vi "zad1.vi"() -> ()   [LabVIEW 2017]
panel:
  out "result string":string[](array[string])
  in  "tekst":string
  in  "litera":string
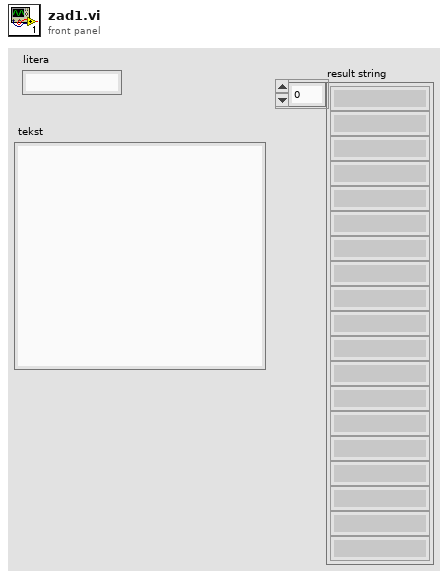
[diagram p1: front panel]
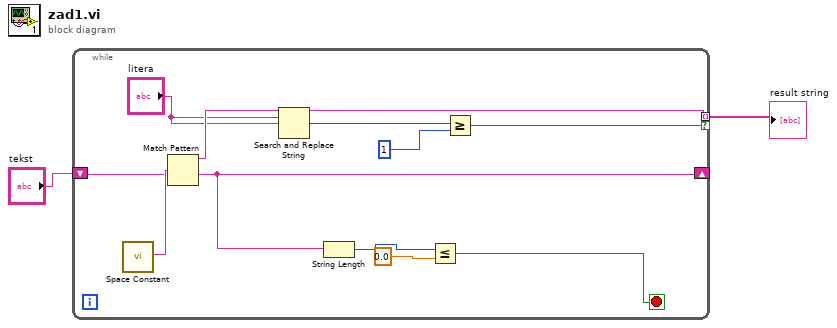
[diagram p0: block diagram]
diagram:
  n1 = while {
    shift-right: [w7] -> _
    shift-left: "tekst" -> [w9]
    tunnel: [w8] -> w1 mode=indexing if=w3
    stop <- w4 stop-if-true
    n2 = call <vilib>:"Space Constant.vi"() -> ("String"=w14:string)
    n3 = Match Pattern(string=w9, regular expression=w14) -> (before substring=w13:string, after substring=w7:string)  [unwired: 1 in, 2 out]
    n4 = Search and Replace String(input string=w13, search string="litera", replace string="litera") -> (result string=w8:string, number of replacements=w11:i32)  [unwired: 5 in, 2 out]
    n5 = String Length(string=w7) -> (length=w5:i32)
    n6 = Less Or Equal?(x=w5, y=0.0) -> (x <= y?=w4:bool)
    n7 = Greater Or Equal?(x=w11, y=1) -> (x >= y?=w3:bool)
  }
  "result string" <- w1
